vi "Actor Core.vi"(8 "error in":errorcluster, 11 "Controller in":refnum<class "Controller.lvclass">) -> (0 "error out":errorcluster, 3 "Actor out":refnum<class "Actor.lvclass">)   [LabVIEW 2015, in "Controller.lvlib" / "Controller.lvclass"]
doc: "(<B>Filename</B>: Actor Framework.lvlib:Actor.lvclass:Actor Core.vi)\n\nReceives messages to the actor, reacts to them, and initiates any error handling that may shut the actor down.\n\nDescendant classes may override this VI to append parallel tasks for the actor to complete while it handles messages. Overrides use the Call Parent Method node."
uses:
  Controller.lvclass
  <vilib>/ActorFramework/Actor/Actor.lvclass
  User Interface/User Interface/User Interface.lvclass
  Database/Database/Database.lvclass
  Hardware/Hardware/Hardware.lvclass
  Database/Database Messages/Open Config File Msg/Open Config File Msg.lvclass/Open Config File Msg.ctl
  <vilib>/ActorFramework/Message Enqueuer/Message Enqueuer.lvclass/Message Enqueuer.ctl
  Controller.lvclass/Controller.ctl
  <vilib>/ActorFramework/Message Enqueuer/Enqueue.vi
  <vilib>/ActorFramework/Message Priority Queue/Priority Enqueue.vi
  Database/Database Messages/Open Config File Msg/Open Config File Msg.lvclass
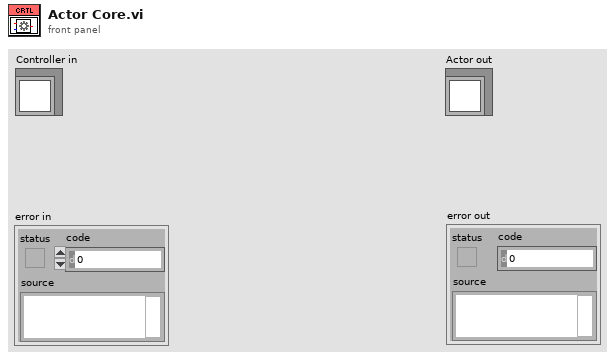
[diagram p1: front panel]
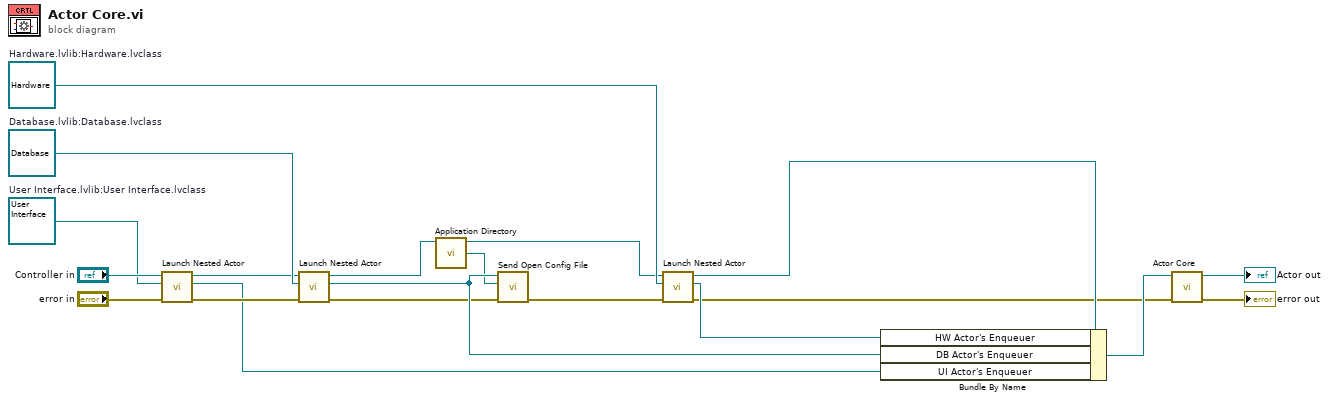
[diagram p0: block diagram]
diagram:
  w13 = refnum<class "Hardware.lvclass"> refnum  # Hardware.lvlib:Hardware.lvclass
  w14 = refnum<class "Database.lvclass"> refnum  # Database.lvlib:Database.lvclass
  w15 = refnum<class "User Interface.lvclass"> refnum  # User Interface.lvlib:User Interface.lvclass
  n1 = call <vilib>:"Launch Nested Actor.vi"("error in (no error)"="error in", "Nested Actor"=w15, "Caller Actor in"="Controller in") -> ("error out"=w11:errorcluster, "Nested Actor's Enqueuer"=w9:refnum<class "Message Enqueuer.lvclass">, "Caller Actor out"=w12:refnum<class "Controller.lvclass">)  [unwired: 6 in]
  n2 = call <vilib>:"Launch Nested Actor.vi"("error in (no error)"=w11, "Nested Actor"=w14, "Caller Actor in"=w12) -> ("error out"=w3:errorcluster, "Nested Actor's Enqueuer"=w5:refnum<class "Message Enqueuer.lvclass">, "Caller Actor out"=w2:refnum<class "Controller.lvclass">)  [unwired: 6 in]
  n3 = call <vilib>:"Application Directory.vi"() -> ("Application Directory"=w4:path)
  n4 = call "Send Open Config File.vi"("error in (no error)"=w3, "Config File Path"=w4, "Message Enqueuer"=w5) -> ("error out"=w1:errorcluster)  [unwired: 7 in, 1 out]
  n5 = call <vilib>:"Launch Nested Actor.vi"("error in (no error)"=w1, "Nested Actor"=w13, "Caller Actor in"=w2) -> ("error out"=w6:errorcluster, "Nested Actor's Enqueuer"=w7:refnum<class "Message Enqueuer.lvclass">, "Caller Actor out"=w10:refnum<class "Controller.lvclass">)  [unwired: 6 in]
  n6 = Bundle By Name(cluster=w10, "HW Actor's Enqueuer"=w7, "DB Actor's Enqueuer"=w5, "UI Actor's Enqueuer"=w9) -> (w8:refnum<class "Controller.lvclass">)
  n7 = call-parent "Actor Core.vi"("error in"=w6, "Actor in"=w8) -> ("error out"=→"error out":errorcluster, "Actor out"=→"Actor out":refnum<class "Actor.lvclass">)  [unwired: 8 in]
